vi "Large integer U8 array - multiply.vi"(3 "Large number - U8 2":T1, 5 "Large number - U8 1":T1) -> (1 "Multiplied array":T1)   [LabVIEW 2013]
doc: "Multiplies two large numbers (U8 array format)."
uses:
  User Access Type defs/Large number - U8 array.ctl
panel:
  # "index 0 = LSD"
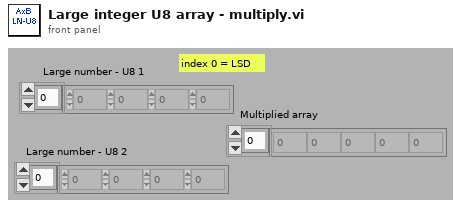
[diagram p1: front panel]
types:
  T1 = typedef "Large number - U8 array.ctl" = u8[]
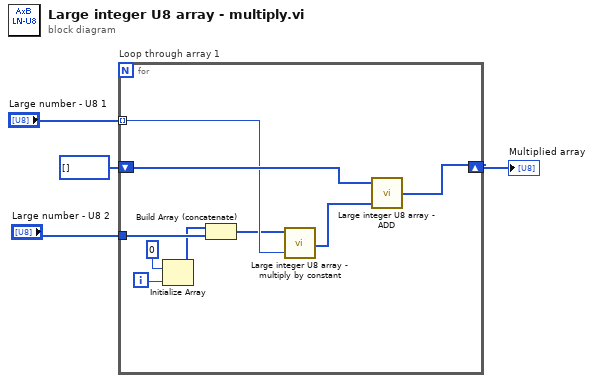
[diagram p0: block diagram]
diagram:
  n1 = for "Loop through array 1" {
    shift-right: [w12] -> w1
    shift-left: T1 [] ("Added array") -> [w13]
    tunnel: "Large number - U8 2" -> [w10]
    tunnel: "Large number - U8 1" -> [w7] mode=indexing
    i -> [w11]
    n2 = Initialize Array(u8 0, w11) -> (w9:u8[])
    n3 = Build Array (concatenate)(w9, w10) -> (w6:T1)
    n4 = call "Large integer U8 array - multiply by constant.vi"("Constant U8"=w7, "Large number - U8"=w6) -> ("Multiplied array"=w5:T1)  [unwired: 3 out]
    n5 = call "Large integer U8 array - ADD.vi"("Large number - U8 2"=w5, "Large number - U8 1"=w13) -> ("Added array"=w12:T1)  [unwired: 3 out]
  }
  "Multiplied array" <- w1
